vi "9402_Initialize.vi"(8 "error in (no error)":errorcluster, 9 "Slot Settings":T1, 11 "9402 in":refnum<class "9402.lvclass">) -> (0 "error out":errorcluster, 3 "9402 out":refnum<class "9402.lvclass">)   [LabVIEW 2017, in "Modules.lvlib" / "9402.lvclass"]
uses:
  9402.lvclass
  RSI Module/Slot Settings.ctl
  C:/Users/dbuck/Documents/GitHub/Scan-Engine-Custom-Device-Classes/Source/SD Module/SD Module.lvclass
  C:/Users/dbuck/Documents/GitHub/Scan-Engine-Custom-Device-Classes/Source/RSI Module/RSI Module.lvclass
  RSI Module/Channels.ctl
  RSI Module/Channel Type.ctl
  RSI Module/Module Models.ctl
  9402.lvclass/9402.ctl
  RSI Module/RSI Module.lvclass
  SD Module/SD Module.lvclass
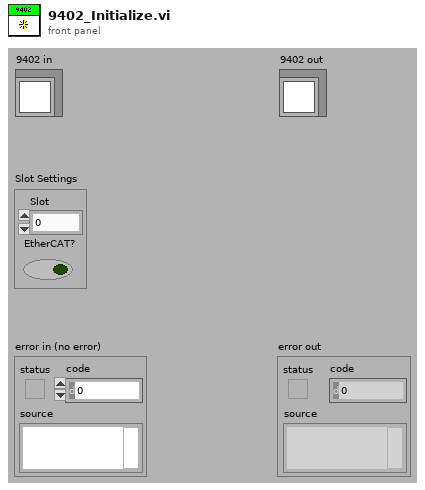
[diagram p1: front panel]
types:
  T1 = typedef "Modules.lvlib/RSI Module.lvclass/Slot Settings.ctl" = cluster{"Slot":u32, "EtherCAT?":bool}
  T2 = typedef "Modules.lvlib/RSI Module.lvclass/Module Models.ctl" = enum16{"Empty", "NI 9201", "NI 9203", "NI 9205", "NI 9206", "NI 9207", "NI 9208", "NI 9211", "NI 9212", "NI 9213", "NI 9214", "NI 9215", "NI 9217", "NI 9219", "NI 9220", "NI 9221", "NI 9222", "NI 9223", "NI 9225", "NI 9227", "NI 9229", "NI 9233", "NI 9234", "NI 9235", "NI 9236", "NI 9237", "NI 9239", "NI 9242", "NI 9244", "NI 9263", "NI 9264", "NI 9265", "NI 9269", "NI 9375", "NI 9401", "NI 9402", "NI 9403", "NI 9411", "NI 9421", "NI 9422", "NI 9423", "NI 9425", "NI 9426", "NI 9435", "NI 9437", "NI 9472", "NI 9474", "NI 9475", "NI 9476", "NI 9477", "NI 9478", "NI 9481", "NI 9482", "NI 9485"}
  T3 = typedef "Modules.lvlib/RSI Module.lvclass/Channels.ctl" = cluster{"# Input Channels":i32, "# Output Channels":i32, "Channel Type":T4, "Units":string}
  T4 = typedef "Modules.lvlib/RSI Module.lvclass/Channel Type.ctl" = enum16{"Analog", "Digital"}
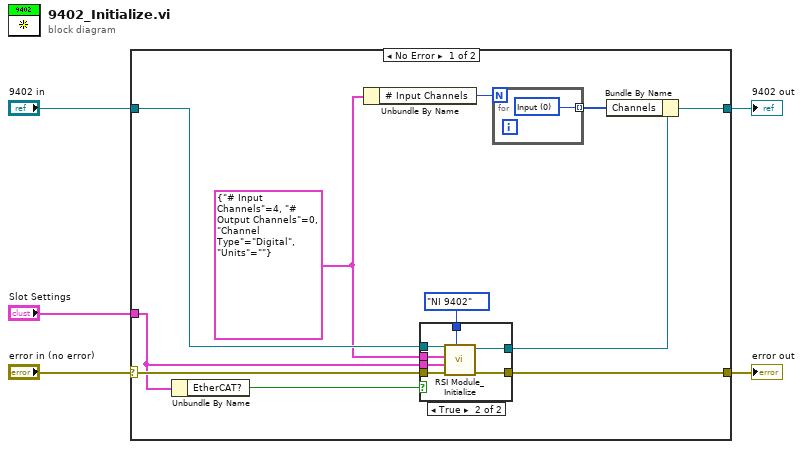
[diagram p0: block diagram]
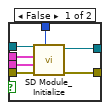
[diagram p2: hidden frame]
diagram:
  n1 = case shown="No Error" "error in (no error)" {
    selector: "error in (no error)" -> [w15 w33]
    tunnel: [w14 w33] -> w4
    tunnel: [w12 w32] -> w2
    tunnel: "9402 in" -> [w16 w32]
    tunnel: "Slot Settings" -> [w7 _]
    frame No Error {
      w9 = T3 {"# Input Channels"=4, "# Output Channels"=0, "Channel Type"=enum."Digital", "Units"=""} ("Channels")
      n2 = Unbundle By Name(w7) -> ("EtherCAT?"=w6:bool)
      n3 = Unbundle By Name(w9) -> ("# Input Channels"=w8:i32)
      n4 = case shown="True" w6 {
        tunnel: w16 -> [w23 w27]
        tunnel: w7 -> [w22 w25]
        tunnel: w15 -> [w21 w26]
        tunnel: [w20 w28] -> w14
        tunnel: [w19 w29] -> w13
        tunnel: Module_Models."NI 9402" ("Module Model") -> [w18 w30]
        tunnel: w9 -> [w17 w24]
        frame False {
          n5 = call "SD Module_Initialize.vi"("Module Model"=w18, "error in (no error)"=w21, "Slot Settings"=w22, "Channels"=w17, "SD Module in"=w23) -> ("error out"=w20:errorcluster, "SD Module out"=w19:refnum<class "9402.lvclass">)  [unwired: 5 in]
        }
        frame True {
          n6 = call "RSI Module_Initialize.vi"("Module Model"=w30, "error in (no error)"=w26, "Slot Settings"=w25, "Channels"=w24, "RSI Module in"=w27) -> ("error out"=w28:errorcluster, "RSI Module out"=w29:refnum<class "9402.lvclass">)  [unwired: 5 in]
        }
      }
      n7 = for {
        N: w8 -> [_]
        tunnel: [w31] -> w10 mode=indexing
        w31 = u32 0 items=["Input", "Output"] ("Line direction")
      }
      n8 = Bundle By Name(cluster=w13, "Channels"=w10) -> (w12:refnum<class "9402.lvclass">)
    }
    frame Error {
    }
  }
  "error out" <- w4
  "9402 out" <- w2
